vi "4_1_power spectrum of signals.vi"() -> ()   [LabVIEW 2009]
uses:
  <vilib>/Analysis/2dsp.llb/Real FFT.vi
  <vilib>/measure/matone.llb/Extract Single Tone Information 1 Chan.vi
  <vilib>/Analysis/NI_AALBase.lvlib
  <vilib>/measure/NI_MAPro.lvlib
  <vilib>/Analysis/NI_AALPro.lvlib
panel:
  out "Entropy":dbl
  out "?":bool
  out "?":bool
  out "DETECTED FREQUENCY":dbl=0.010000000000000035 format="%.2p"
  out "POWER SPECTRUM":cluster{i32, dbl, dbl[]}(graph)={0, 10.0, [8.485769562298236e-31, 0.49999999999999944, 8.164307715079776e-31, 3.3743626163259144e-31, 1.825019551236016e-31, 7.402762362304142e-32, 4.2710856054145054e-32, 4.1564672555215647e-32, 2.6702087071432447e-32, 2.4623303346019908e-32, 1.6389617625607408e-32, 7.677570627885547e-33, 1.239492669969223e-32, 8.411277506077035e-33, 9.078916870112728e-33, 8.640859019051572e-33, 6.176660695964688e-33, 6.952762004088197e-33, 5.4024269896079905e-33, 6.8532456269935766e-34, 4.903901452689594e-33, 1.2323312743318063e-32, 4.3025523760552065e-33, 4.61657185236404e-33, 3.737037046365132e-33, 2.9304844668360058e-33, 3.0127672679888278e-33, 2.5999745698237937e-33, 3.621228144408738e-33, 6.993769099327424e-33, 2.3516648842844825e-33, 7.462680110760539e-34, 2.2202019748107235e-33, 1.9910882800103614e-33, 2.0841511415246487e-33, 2.3785746525111287e-33, 2.105843427884887e-33, 1.821930903521826e-33, 2.046515420923481e-33, 3.2148901133684515e-33, 1.7488258575267894e-33, 3.359262437668602e-33, 1.72433666249381e-33, 1.778603419745664e-33, 1.4624219142263041e-33, 1.5783345443116216e-33, 2.2614347719326688e-33, 1.4283574382420044e-33, 1.5348234654298793e-33, 3.720876456897524e-33]}
  out "# OF CYCLES":dbl=1.0
  in  "?":bool
  out "?":string="Sample"
  out "PERIODIC REPETITION":dbl[](graph)=[0.0, 0.06279051952931337, 0.12533323356430426, 0.18738131458572463, 0.2486898871648548, 0.3090169943749474, 0.368124552684678, 0.42577929156507266, 0.4817536741017153, 0.5358267949789967, 0.5877852522924732, 0.6374239897486899, 0.6845471059286888, 0.7289686274214117, 0.7705132427757894, 0.8090169943749476, 0.8443279255020152, 0.8763066800438637, 0.9048270524660196, 0.9297764858882515, 0.9510565162951535, 0.9685831611286311, 0.9822872507286886, 0.9921147013144778, 0.9980267284282716, 1.0, 0.9980267284282716, 0.9921147013144779, 0.9822872507286888, 0.9685831611286313, 0.9510565162951539, 0.9297764858882518, 0.90482705246602, 0.8763066800438643, 0.8443279255020159, 0.8090169943749483, 0.7705132427757903, 0.7289686274214127, 0.6845471059286901, 0.6374239897486912, 0.5877852522924748, 0.5358267949789984, 0.4817536741017172, 0.42577929156507477, 0.3681245526846802, 0.30901699437494984, 0.24868988716485732, 0.18738131458572732, 0.12533323356430706, 0.0627905195293163, 3.0294235002503722e-15, -0.06279051952931025, -0.12533323356430104, -0.18738131458572135, -0.24868988716485146, -0.30901699437494407, -0.3681245526846746, -0.4257792915650693, -0.48175367410171194, -0.5358267949789933, -0.5877852522924699, -0.6374239897486865, -0.6845471059286856, -0.7289686274214086, -0.7705132427757864, -0.8090169943749448, -0.8443279255020126, -0.8763066800438613, -0.9048270524660175, -0.9297764858882496, -0.951056516295152, -0.9685831611286299, -0.9822872507286877, -0.9921147013144772, -0.9980267284282713, -1.0, -0.9980267284282718, -0.9921147013144782, -0.9822872507286892, -0.9685831611286317, -0.9510565162951542, -0.929776485888252, -0.90482705246602, -0.876306680043864, -0.8443279255020153, -0.8090169943749475, -0.770513242775789, -0.728968627421411, -0.6845471059286878, -0.6374239897486885, -0.5877852522924716, -0.5358267949789947, -0.48175367410171294, -0.4257792915650699, -0.36812455268467476, -0.30901699437494373, -0.24868988716485066, -0.18738131458572005, -0.12533323356429923, -0.06279051952930793, 0.0, 0.06279051952931337, 0.12533323356430426, 0.18738131458572463, 0.2486898871648548, 0.3090169943749474, 0.368124552684678, 0.42577929156507266, 0.4817536741017153, 0.5358267949789967, 0.5877852522924732, 0.6374239897486899, 0.6845471059286888, 0.7289686274214117, 0.7705132427757894, 0.8090169943749476, 0.8443279255020152, 0.8763066800438637, 0.9048270524660196, 0.9297764858882515, 0.9510565162951535, 0.9685831611286311, 0.9822872507286886, 0.9921147013144778, 0.9980267284282716, 1.0, 0.9980267284282716, 0.9921147013144779, 0.9822872507286888, 0.9685831611286313, 0.9510565162951539, 0.9297764858882518, 0.90482705246602, 0.8763066800438643, 0.8443279255020159, 0.8090169943749483, 0.7705132427757903, 0.7289686274214127, 0.6845471059286901, 0.6374239897486912, 0.5877852522924748, 0.5358267949789984, 0.4817536741017172, 0.42577929156507477, 0.3681245526846802, 0.30901699437494984, 0.24868988716485732, 0.18738131458572732, 0.12533323356430706, 0.0627905195293163, 3.0294235002503722e-15, -0.06279051952931025, -0.12533323356430104, -0.18738131458572135, -0.24868988716485146, -0.30901699437494407, -0.3681245526846746, -0.4257792915650693, -0.48175367410171194, -0.5358267949789933, -0.5877852522924699, -0.6374239897486865, -0.6845471059286856, -0.7289686274214086, -0.7705132427757864, -0.8090169943749448, -0.8443279255020126, -0.8763066800438613, -0.9048270524660175, -0.9297764858882496, -0.951056516295152, -0.9685831611286299, -0.9822872507286877, -0.9921147013144772, -0.9980267284282713, -1.0, -0.9980267284282718, -0.9921147013144782, -0.9822872507286892, -0.9685831611286317, -0.9510565162951542, -0.929776485888252, -0.90482705246602, -0.876306680043864, -0.8443279255020153, -0.8090169943749475, -0.770513242775789, -0.728968627421411, -0.6845471059286878, -0.6374239897486885, -0.5877852522924716, -0.5358267949789947, -0.48175367410171294, -0.4257792915650699, -0.36812455268467476, -0.30901699437494373, -0.24868988716485066, -0.18738131458572005, -0.12533323356429923, -0.06279051952930793]
  out "ORIGINAL SIGNAL":T1(graph)={0, "# OF SAMPLES"=1.0, "Sinc Pattern"=[0.0, 0.06279051952931337, 0.12533323356430426, 0.18738131458572463, 0.2486898871648548, 0.3090169943749474, 0.368124552684678, 0.42577929156507266, 0.4817536741017153, 0.5358267949789967, 0.5877852522924732, 0.6374239897486899, 0.6845471059286888, 0.7289686274214117, 0.7705132427757894, 0.8090169943749476, 0.8443279255020152, 0.8763066800438637, 0.9048270524660196, 0.9297764858882515, 0.9510565162951535, 0.9685831611286311, 0.9822872507286886, 0.9921147013144778, 0.9980267284282716, 1.0, 0.9980267284282716, 0.9921147013144779, 0.9822872507286888, 0.9685831611286313, 0.9510565162951539, 0.9297764858882518, 0.90482705246602, 0.8763066800438643, 0.8443279255020159, 0.8090169943749483, 0.7705132427757903, 0.7289686274214127, 0.6845471059286901, 0.6374239897486912, 0.5877852522924748, 0.5358267949789984, 0.4817536741017172, 0.42577929156507477, 0.3681245526846802, 0.30901699437494984, 0.24868988716485732, 0.18738131458572732, 0.12533323356430706, 0.0627905195293163, 3.0294235002503722e-15, -0.06279051952931025, -0.12533323356430104, -0.18738131458572135, -0.24868988716485146, -0.30901699437494407, -0.3681245526846746, -0.4257792915650693, -0.48175367410171194, -0.5358267949789933, -0.5877852522924699, -0.6374239897486865, -0.6845471059286856, -0.7289686274214086, -0.7705132427757864, -0.8090169943749448, -0.8443279255020126, -0.8763066800438613, -0.9048270524660175, -0.9297764858882496, -0.951056516295152, -0.9685831611286299, -0.9822872507286877, -0.9921147013144772, -0.9980267284282713, -1.0, -0.9980267284282718, -0.9921147013144782, -0.9822872507286892, -0.9685831611286317, -0.9510565162951542, -0.929776485888252, -0.90482705246602, -0.876306680043864, -0.8443279255020153, -0.8090169943749475, -0.770513242775789, -0.728968627421411, -0.6845471059286878, -0.6374239897486885, -0.5877852522924716, -0.5358267949789947, -0.48175367410171294, -0.4257792915650699, -0.36812455268467476, -0.30901699437494373, -0.24868988716485066, -0.18738131458572005, -0.12533323356429923, -0.06279051952930793]}
  in  "stop":bool
  in  "Delta t":dbl=0.1 format="%0.2f"
  in  "Duty cycle (%)":dbl=50.0 format="%0.2f"
  in  "Width":i32=1
  in  "Start":dbl format="%0.2f"
  in  "End":dbl=1.0 format="%0.2f"
  in  "Reset phase":bool=TRUE
  in  "DELAY":dbl(knob) min=0.0 max=10.0 scale=0.0..10.0
  in  "AMPLITUDE":dbl=1.0
  in  "PHASE IN":dbl(knob) scale=0.0..180.0
  in  "SIGNAL FREQUENCY":dbl(knob)=10.0 scale=0.0..10000.0 scale format="%#_6p"
  in  "SAMPLING\nFREQUENCY (Hz)":dbl(slide)=1000.0 scale=0.0..20000.0 scale format="%#_6p"
  in  "# OF SAMPLES":dbl=100.0
  in  "SIGNAL":T2(ring)
  # "Program developed by Indranil Sinharoy"
  # "ORIGINAL SIGNAL \nCHARACTERISTICS"
  # "RAMP"
  # "PULSE"
  # "SQUARE"
  # "SINC"
  # "SAMPLING INFO"
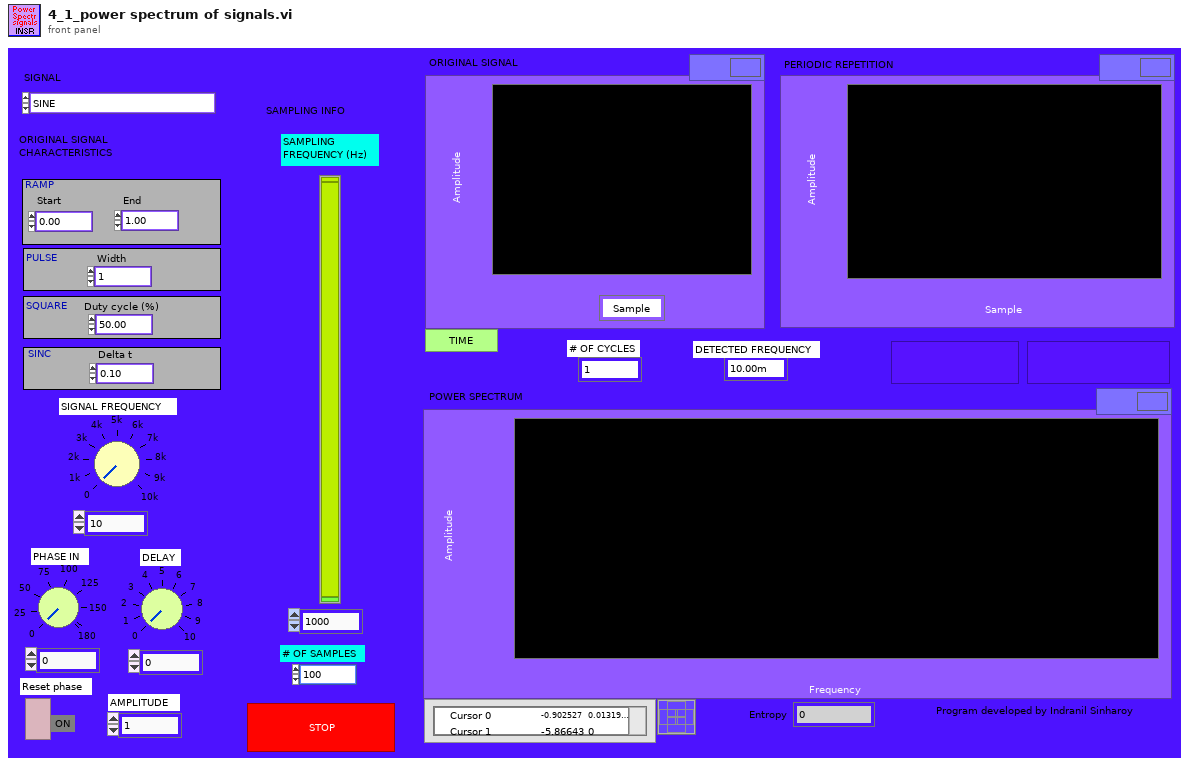
[diagram p1: front panel]
types:
  T1 = cluster{i32, "# OF SAMPLES":dbl, "Sinc Pattern":dbl[]}
  T2 = enum16{"SINE", "TRIANGULAR", "RAMP", "IMPULSE", "SINC ", "PULSE", "SQUARE"}
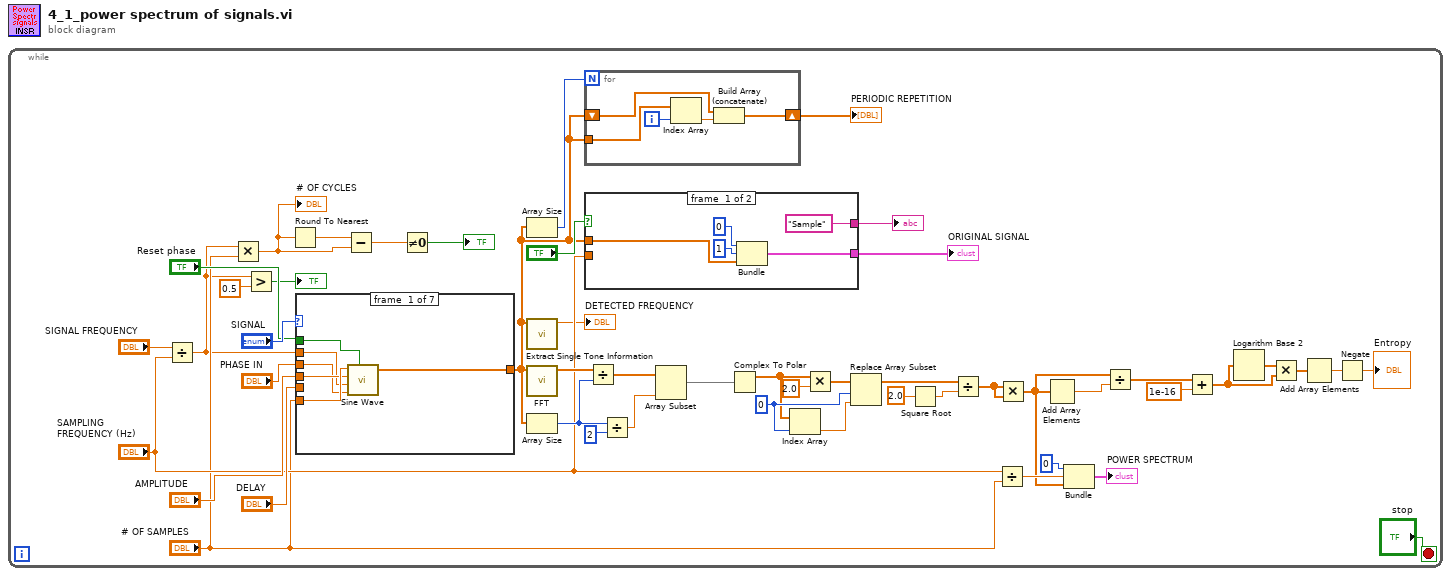
[diagram p0: block diagram]
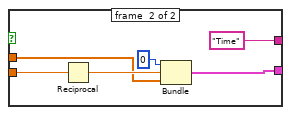
[diagram p2: hidden frame]
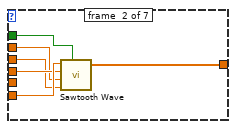
[diagram p3: hidden frame]
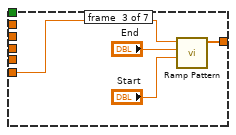
[diagram p4: hidden frame]
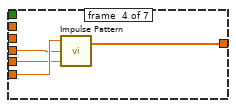
[diagram p5: hidden frame]
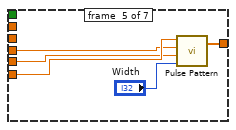
[diagram p6: hidden frame]
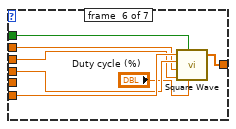
[diagram p7: hidden frame]
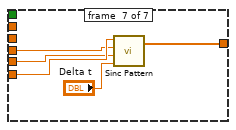
[diagram p8: hidden frame]
diagram:
  n1 = while {
    stop <- "stop" stop-if-true
    w34 = 0 ("index")
    n2 = Divide(x="SIGNAL FREQUENCY", y="SAMPLING\nFREQUENCY (Hz)") -> (x/y=w15:dbl)
    n3 = Multiply(x=w15, y="# OF SAMPLES") -> (x*y=w12:dbl)
    "# OF CYCLES" <- w12
    n4 = Greater?(x=w15, y=0.5) -> (0:→"?":bool)
    n5 = Round To Nearest(number=w12) -> (nearest integer value=w13:dbl)
    n6 = case shown="\"RAMP\"" "SIGNAL" {
      tunnel: "Reset phase" -> [w72 w78 _ _ _ w98 _]
      tunnel: "AMPLITUDE" -> [w70 w76 _ w85 w90 w96 w102]
      tunnel: "# OF SAMPLES" -> [w71 w77 w81 w86 w91 w97 w103]
      tunnel: w15 -> [w69 w75 _ _ _ w95 _]
      tunnel: "PHASE IN" -> [w68 w74 _ _ _ w94 _]
      tunnel: "DELAY" -> [_ _ _ w84 w89 _ w101]
      tunnel: [w67 w73 w82 w83 w88 w93 w100] -> w21
      frame #0 {
        n7 = call <vilib>:"Sine Wave.vi"("samples"=w71, "amplitude"=w70, "frequency"=w69, "phase in"=w68, "reset phase"=w72) -> ("sine wave"=w67:dbl[])  [unwired: 2 out]
      }
      frame #1 {
        n8 = call <vilib>:"Sawtooth Wave.vi"("samples"=w77, "amplitude"=w76, "frequency"=w75, "phase in"=w74, "reset phase"=w78) -> ("sawtooth wave"=w73:dbl[])  [unwired: 2 out]
      }
      frame #2 {
        n9 = call <vilib>:"Ramp Pattern.vi"("start"="Start", "end"="End", "samples"=w81) -> ("Ramp Pattern"=w82:dbl[])  [unwired: 7 in, 1 out]
      }
      frame #3 {
        n10 = call <vilib>:"Impulse Pattern.vi"("delay"=w84, "amplitude"=w85, "samples"=w86) -> ("Impulse Pattern"=w83:dbl[])  [unwired: 1 out]
      }
      frame #4 {
        n11 = call <vilib>:"Pulse Pattern.vi"("width"="Width", "delay"=w89, "amplitude"=w90, "samples"=w91) -> ("Pulse Pattern"=w88:dbl[])  [unwired: 1 out]
      }
      frame #5 {
        n12 = call <vilib>:"Square Wave.vi"("samples"=w97, "reset phase"=w98, "amplitude"=w96, "frequency"=w95, "duty cycle (%)"="Duty cycle (%)", "phase in"=w94) -> ("square wave"=w93:dbl[])  [unwired: 2 out]
      }
      frame #6 {
        n13 = call <vilib>:"Sinc Pattern.vi"("delta t"="Delta t", "delay"=w101, "amplitude"=w102, "samples"=w103) -> ("Sinc Pattern"=w100:dbl[])  [unwired: 1 out]
      }
    }
    n14 = Subtract(x=w13, y=w12) -> (x-y=w11:dbl)
    n15 = Not Equal To 0?(x=w11) -> (x != 0?=→"?":bool)
    n16 = Array Size(array=w21) -> (size(s)=w42:i32)
    n17 = call-poly <vilib>:"Extract Single Tone Information.vi"("time signal in"=w21) -> ("detected frequency"=→"DETECTED FREQUENCY":dbl)  [unwired: 5 in, 5 out]
    n18 = call-poly <vilib>:"FFT.vi"("X"=w21) -> ("FFT {X}"=w41:cdb[])  [unwired: 9 in, 1 out]
    n19 = Array Size(array=w21) -> (size(s)=w38:i32)
    n20 = for {
      N: w42 -> [_]
      shift-right: [w54] -> w18
      shift-left: w21 -> [w53]
      tunnel: w21 -> [w51]
      i -> [w52]
      n21 = Index Array(array=w51, index=w52) -> (element=w55:dbl)
      n22 = Build Array (concatenate)(w53, w55) -> (w54:dbl[])
    }
    "PERIODIC REPETITION" <- w18
    n23 = case shown="True" "?" {
      tunnel: w21 -> [w59 w64]
      tunnel: [w57 w62] -> w43
      tunnel: "SAMPLING\nFREQUENCY (Hz)" -> [_ w66]
      tunnel: ["Sample" "Time"] -> w17
      frame #0 {
        n24 = Bundle(0, 1, "Sinc Pattern"=w59) -> (w57:cluster{i32, i32, "Sinc Pattern":dbl[]})  [unwired: 1 in]
      }
      frame #1 {
        n25 = Reciprocal(x=w66) -> (1/x=w65:dbl)
        n26 = Bundle(0, w65, "Sinc Pattern"=w64) -> (w62:cluster{i32, dbl, "Sinc Pattern":dbl[]})  [unwired: 1 in]
      }
    }
    "ORIGINAL SIGNAL" <- w43
    "?" <- w17
    n27 = Divide(x=w41, y=w38) -> (x/y=w40:cdb[])
    n28 = Divide(x=w38, y=2) -> (x/y=w39:dbl)
    n29 = Array Subset(array=w40, length=w39) -> (w36:cdb[])  [unwired: 1 in]
    n30 = Complex To Polar(r * e^(i*theta)=w36) -> (r=w32:dbl[])  [unwired: 1 out]
    n31 = Index Array(array=w32, index=w34) -> (element=w35:dbl)
    n32 = Multiply(x=w32, y=2.0) -> (x*y=w33:dbl[])
    n33 = Replace Array Subset(array=w33, new element=w35, index=w34) -> (w30:dbl[])
    n34 = Square Root(x=2.0) -> (sqrt(x)=w29:dbl)
    n35 = Divide(x=w30, y=w29) -> (x/y=w27:dbl[])
    n36 = Divide(x="SAMPLING\nFREQUENCY (Hz)", y="# OF SAMPLES") -> (x/y=w23:dbl)
    n37 = Multiply(x=w27, y=w27) -> (x*y=w5:dbl[])
    n38 = Add Array Elements(numeric array=w5) -> (sum=w4:dbl)
    n39 = Bundle(0, w23, w5) -> (→"POWER SPECTRUM":cluster{i32, dbl, dbl[]})  [unwired: 1 in]
    n40 = Divide(x=w5, y=w4) -> (x/y=w3:dbl[])
    n41 = Add(x=w3, y=1e-16) -> (x+y=w2:dbl[])
    n42 = Logarithm Base 2(1:w2) -> (0:w9:dbl[])
    n43 = Multiply(x=w9, y=w2) -> (x*y=w8:dbl[])
    n44 = Add Array Elements(numeric array=w8) -> (sum=w7:dbl)
    n45 = Negate(x=w7) -> (-x=→"Entropy":dbl)
  }
